vi "test Get Set APU.vi"(8 "error in (no error)":errorcluster, 11 "TestCase in":refnum<class "Scripting API Test Case.lvclass">) -> (0 "error out":errorcluster, 3 "TestCase out":refnum<class "Scripting API Test Case.lvclass">)   [LabVIEW 2019, in "Scripting API Test Case.lvclass"]
uses:
  Scripting API Test Case.lvclass
  Scripting API/Custom Device/Engine Simulation Toolkit Custom Device Settings.ctl
  Scripting API/Bitfile/Bitfile.ctl
  Scripting API/APU/APU Settings.ctl
  Scripting API Test Case.lvclass/Scripting API Test Case.ctl
  <userlib>/_OpenG.lib/file/file.llb/Append Path to Root if Relative - Scalar__ogtk.vi
  <vilib>/addons/_JKI Toolkits/VI Tester/TestCase.llb/TestCase.lvclass
  niveristand-custom-device-testing-tools/VeriStandTestUtilities/VeriStandTestUtilities.lvlib
  Scripting API/Engine Simulation Toolkit Scripting API.lvlib
  C:/Program Files (x86)/National Instruments/LabVIEW 2019/vi.lib/addons/_JKI Toolkits/VI Tester/TestCase.llb/TestCase.lvclass
panel:
  in  "Save?":bool
  out "Output Filename":string
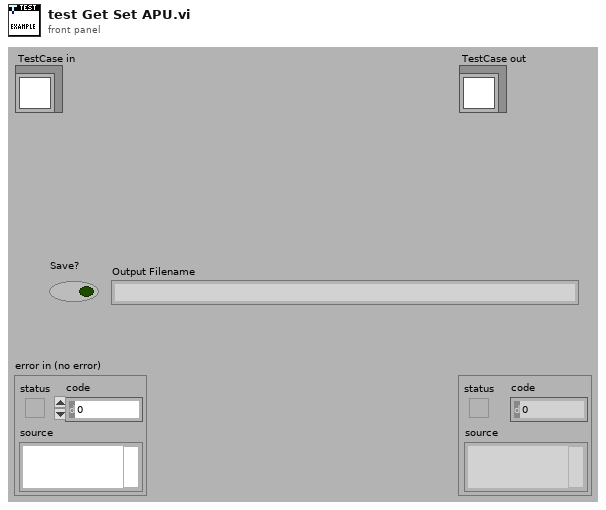
[diagram p1: front panel]
types:
  T1 = typedef "Engine Simulation Toolkit Scripting API.lvlib/Bitfile.ctl" = cluster{"RIO Device Address":string, "Bitfile Path":path}
  T2 = typedef "Engine Simulation Toolkit Scripting API.lvlib/Engine Simulation Toolkit Custom Device Settings.ctl" = cluster{"Name":string, "Execution priority":enum16{"Low", "Medium", "High"}, "Rate decimation":i32, "CPU":i32}
  T3 = typedef "Engine Simulation Toolkit Scripting API.lvlib/APU Settings.ctl" = cluster{"Name":string, "Start angle (degrees)":dbl, "des speed":dbl, "Acceleration":bool, "des accel":dbl, "Maximum angle deviation\nbetween RIO devices (degrees)":dbl}
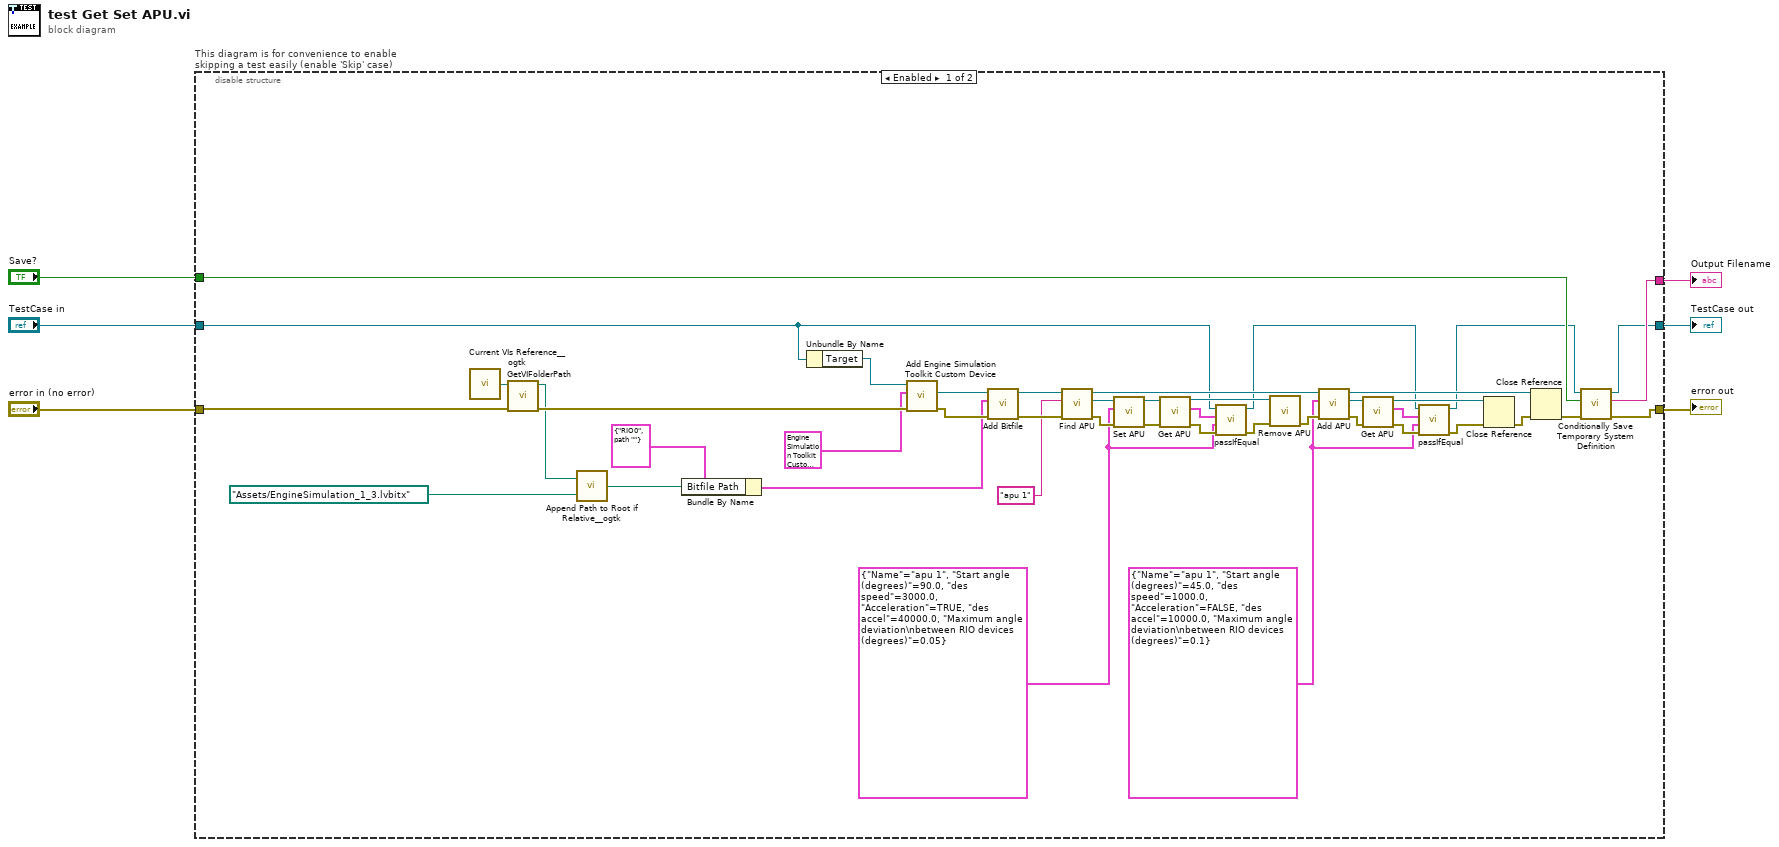
[diagram p0: block diagram]
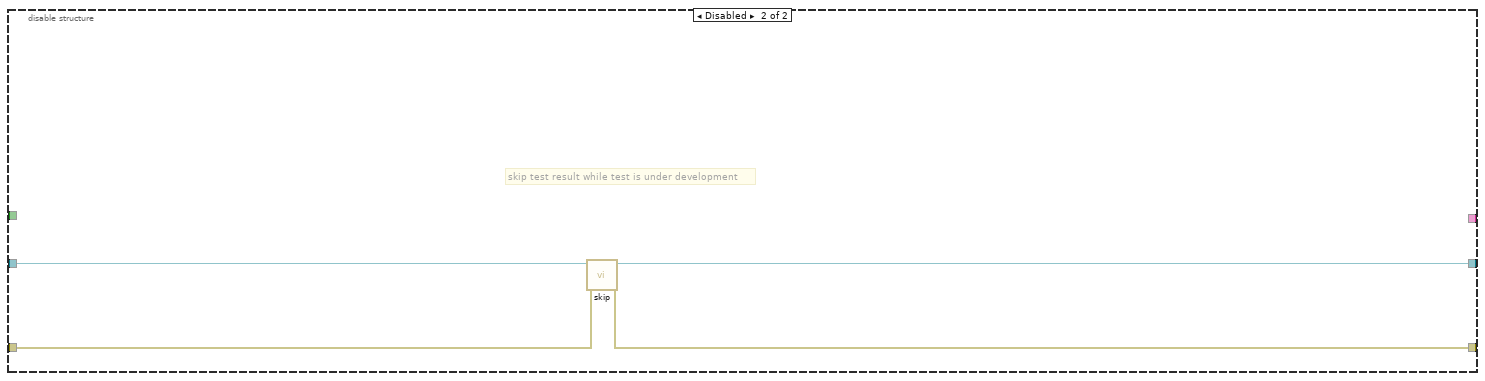
[diagram p2: hidden frame]
diagram:
  n1 = disable-structure "This diagram is for convenience to enable skipping a test easily (enable 'Skip' case)" shown="Enabled" {
    disable-tunnel: "TestCase in" -> [w8 w53]
    disable-tunnel: [w9 w51] -> w3
    disable-tunnel: [w45 w52] -> w5
    disable-tunnel: "error in (no error)" -> [w48 w50]
    disable-tunnel: [w44 _] -> w2
    disable-tunnel: "Save?" -> [w43 _]
    frame Enabled {
      w15 = T3 {"Name"="apu 1", "Start angle (degrees)"=45.0, "des speed"=1000.0, "Acceleration"=FALSE, "des accel"=10000.0, "Maximum angle deviation\nbetween RIO devices (degrees)"=0.1} ("APU Settings")
      w24 = T3 {"Name"="apu 1", "Start angle (degrees)"=90.0, "des speed"=3000.0, "Acceleration"=TRUE, "des accel"=40000.0, "Maximum angle deviation\nbetween RIO devices (degrees)"=0.05} ("APU Settings")
      n2 = call <userlib>:"Current VIs Reference__ogtk.vi"() -> ("Current VI's reference"=w49:refnum<vi>)  [unwired: 5 in]
      n3 = call "GetVIFolderPath.vi"("error in (no error)"=w48, "VI Reference in"=w49) -> ("error out"=w47:errorcluster, "VI Folder Path out"=w39:path)  [unwired: 8 in]
      n4 = call-poly <userlib>:"Append Path to Root if Relative__ogtk.vi"("Absolute or Relative Path"=path "Assets/EngineSimulation_1_3.lvbitx", "Root Path"=w39) -> ("Absolute or Appended Path"=w35:path)
      n5 = Bundle By Name(cluster=T1 {"RIO Device Address"="RIO0", "Bitfile Path"=path ""} ("Engine Simulation Toolkit Bitfile"), "Bitfile Path"=w35) -> (w36:T1)
      n6 = Unbundle By Name(w8) -> ("Target"=w7:refnum<k24>)
      n7 = call "Add Engine Simulation Toolkit Custom Device.vi"("error in (no error)"=w47, "Settings"=T2 {"Name"="Engine Simulation Toolkit Custom Device", "Execution priority"=enum."Medium", "Rate decimation"=1, "CPU"=-2} ("Engine Simulation Toolkit Custom Device Settings"), "Target in"=w7) -> ("error out"=w40:errorcluster, "EST Custom Device"=w42:refnum<k24>)  [unwired: 6 in, 1 out]
      n8 = call "Add Bitfile.vi"("error in (no error)"=w40, "Engine Simulation Toolkit Bitfile"=w36, "EST Custom Device in"=w42) -> ("error out"=w33:errorcluster, "EST Custom Device out"=w34:refnum<k24>)  [unwired: 7 in]
      n9 = call "Find APU.vi"("error in (no error)"=w33, "Name"="apu 1", "EST Custom Device in"=w34) -> ("error out"=w27:errorcluster, "APU"=w30:refnum<k24>, "EST Custom Device out"=w21:refnum<k24>)  [unwired: 6 in]
      n10 = call "Set APU.vi"("error in (no error)"=w27, "APU Settings"=w24, "APU in"=w30) -> ("error out"=w28:errorcluster, "APU out"=w29:refnum<k24>)  [unwired: 7 in]
      n11 = call "Get APU.vi"("error in (no error)"=w28, "APU in"=w29) -> ("error out"=w26:errorcluster, "APU Settings"=w25:T3, "APU out"=w23:refnum<k24>)  [unwired: 7 in]
      n12 = call-dynamic "passIfEqual.vi"("error in (no error)"=w26, "y"=w24, "x"=w25, "TestCase in"=w8) -> ("error out"=w22:errorcluster, "TestCase out"=w11:refnum<class "Scripting API Test Case.lvclass">)  [unwired: 6 in]
      n13 = call "Remove APU.vi"("error in (no error)"=w22, "APU"=w23) -> ("error out"=w20:errorcluster)  [unwired: 9 in]
      n14 = call "Add APU.vi"("error in (no error)"=w20, "APU Settings"=w15, "EST Custom Device in"=w21) -> ("error out"=w16:errorcluster, "APU"=w17:refnum<k24>, "EST Custom Device out"=w13:refnum<k24>)  [unwired: 6 in]
      n15 = call "Get APU.vi"("error in (no error)"=w16, "APU in"=w17) -> ("error out"=w19:errorcluster, "APU Settings"=w18:T3, "APU out"=w12:refnum<k24>)  [unwired: 7 in]
      n16 = call-dynamic "passIfEqual.vi"("error in (no error)"=w19, "y"=w15, "x"=w18, "TestCase in"=w11) -> ("error out"=w14:errorcluster, "TestCase out"=w10:refnum<class "Scripting API Test Case.lvclass">)  [unwired: 6 in]
      n17 = Close Reference(reference=w12, error in (no error)=w14) -> (error out=w31:errorcluster)
      n18 = Close Reference(reference=w13, error in (no error)=w31) -> (error out=w46:errorcluster)
      n19 = call "Conditionally Save Temporary System Definition.vi"("error in (no error)"=w46, "Save?"=w43, "Test Case"=w10) -> ("error out"=w45:errorcluster, "filename"=w44:string, "Test Case"=w9:refnum<class "Scripting API Test Case.lvclass">)  [unwired: 6 in]
    }
    frame Disabled {
      # "skip test result while test is under development"
      n20 = call <vilib>:"skip.vi"("error in (no error)"=w50, "TestCase in"=w53) -> ("error out"=w52:errorcluster, "TestCase out"=w51:refnum<class "Scripting API Test Case.lvclass">)  [unwired: 8 in]
    }
  }
  "error out" <- w5
  "TestCase out" <- w3
  "Output Filename" <- w2
